vi "AddSequenceRun.vi"(6 "SequenceExecutionStatus (NOT_COMPLETED)":T1=enum."NOT_COMPLETED", 7 "StartDate (Now)":timestamp, 8 "error in":errorcluster, 9 "StationFullName (This Machine)":string, 10 "SequenceFullName":string, 11 "OperationRun in":refnum<class "OperationRun.lvclass">) -> (0 "error out":errorcluster, 2 "SequenceRun":refnum<class "SequenceRun.lvclass">, 3 "OperationRun out":refnum<class "OperationRun.lvclass">)   [LabVIEW 2021, in "ProligentXMLGenerator.lvlib" / "OperationRun.lvclass"]
doc: "Add an OperationRun.\n\nDefines the operation run, a logical container for the execution of sequences and processes.\nOperation runs are globaly unique by their OperationRunId property."
uses:
  OperationRun.lvclass
  OperationRun.lvclass/OperationRun.ctl
  SequenceRun/SequenceRun/SequenceRun.lvclass
  ProligentXMLGenerator.lvlib
  Base/ExecutionStatus/Value.ctl
  Base/ExecutionStatus/ExecutionStatus.lvclass
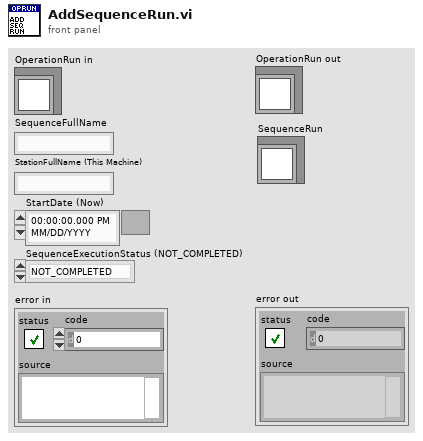
[diagram p1: front panel]
types:
  T1 = typedef "ProligentXMLGenerator.lvlib/ExecutionStatus.lvclass/Value.ctl" = enum16{"PASS", "FAIL", "NOT_COMPLETED", "ABORTED"}
  T2 = typedef "ProligentXMLGenerator.lvlib/OperationRun.lvclass/Data.ctl" = cluster{"Name":string, "Characteristics":refnum<class "Characteristic.lvclass">[], "Documents":refnum<class "Document.lvclass">[], "SequenceRuns":refnum<class "SequenceRun.lvclass">[], "FailureReferences":refnum<class "FailureReference.lvclass">[], "SequenceRunReferences":refnum<class "SequenceRunReference.lvclass">[], "CustomData":refnum<class "CustomData.lvclass">, "OperationRunId":refnum<class "Guid.lvclass">, "ProcessFullName":refnum<class "ProcessFullName.lvclass">, "ProcessVersion":refnum<class "NonEmptyString_64.lvclass">, "OperationName":refnum<class "NonEmptyString_65.lvclass">, "StationFullName":refnum<class "FullName.lvclass">, "User":refnum<class "NonEmptyString_255.lvclass">, "CallingOperationRunId":refnum<class "Guid.lvclass">, "OperationStatus":refnum<class "ExecutionStatus.lvclass">, "OperationRunStartTime":refnum<class "DateTime.lvclass">, "OperationRunEndTime":refnum<class "DateTime.lvclass">, "TimeZoneInfoId":string}
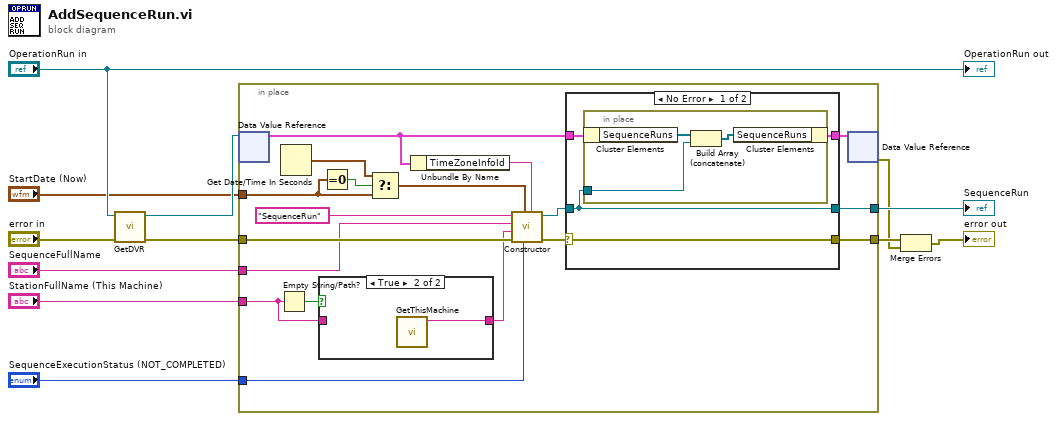
[diagram p0: block diagram]
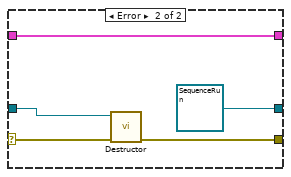
[diagram p3: hidden frame]
diagram:
  n1 = call "GetDVR.vi"("error in"="error in", "OperationRun"="OperationRun in") -> ("error out"=w5:errorcluster, "DVRReference"=w4:refnum<data-value>)  [unwired: 8 in]
  n2 = in-place "In Place Element Structure" {
    in-place-border: "SequenceFullName" -> [w18]
    in-place-border: [w29] -> w6
    in-place-border: w5 -> [w28]
    in-place-border: [w26] -> w8
    in-place-border: "SequenceExecutionStatus (NOT_COMPLETED)" -> [w24]
    in-place-border: "StationFullName (This Machine)" -> [w16]
    in-place-border: "StartDate (Now)" -> [w20]
    n3 = in-place-dvr #1(w4) -> (w14:T2)  [unwired: 1 out]
    n4 = Empty String/Path?(string/path=w16) -> (empty?=w17:bool)
    n5 = Get Date/Time In Seconds() -> (seconds since 1Jan1904=w21:timestamp)
    n6 = case shown="True" w17 {
      tunnel: w16 -> [w31 _]
      tunnel: [w31 w32] -> w15
      frame False {
      }
      frame True {
        n7 = call "GetThisMachine.vi"() -> ("ThisMachine"=w32:string)  [unwired: 11 in]
      }
    }
    n8 = Equal To 0?(x=w20) -> (x = 0?=w22:bool)
    n9 = Select(t=w21, s=w22, f=w20) -> (s? t:f=w19:timestamp)
    n10 = Unbundle By Name(w14) -> ("TimeZoneInfoId"=w13:string)
    n11 = call "Constructor.vi"("TimeZoneInfoId"=w13, "SequenceExecutionStatus"=w24, "StartDate"=w19, "error in"=w28, "StationFullName"=w15, "SequenceFullName"=w18, "Name"="SequenceRun") -> ("error out"=w30:errorcluster, "SequenceRun out"=w25:refnum<class "SequenceRun.lvclass">)  [unwired: 3 in]
    n12 = case shown="No Error" w30 {
      selector: w30 -> [w36 w43]
      tunnel: [w33 w44] -> w27
      tunnel: [w36 w42] -> w29
      tunnel: w25 -> [w35 w41]
      tunnel: w14 -> [w34 w44]
      tunnel: [w35 refnum<class "SequenceRun.lvclass"> refnum ("ProligentResultProcessor:SequenceRun")] -> w26
      frame No Error {
        n13 = in-place "In Place Element Structure" {
          in-place-border: w35 -> [w39]
          n14 = in-place-cluster #2(w34) -> ("SequenceRuns"=w38:refnum<class "SequenceRun.lvclass">[])
          n15 = Build Array (concatenate)(w38, w39) -> (w37:refnum<class "SequenceRun.lvclass">[])
          n16 = in-place-cluster #2("SequenceRuns"=w37) -> (w33:T2)
        }
      }
      frame Error {
        n17 = call "Destructor.vi"("error in"=w43, "SequenceRun"=w41) -> ("error out"=w42:errorcluster)  [unwired: 9 in]
      }
    }
    n18 = in-place-dvr #1(w27) -> (w3:errorcluster)  [unwired: 1 out]
  }
  "SequenceRun" <- w8
  n19 = Merge Errors(w6, w3) -> (→"error out":errorcluster)
  "OperationRun out" <- "OperationRun in"
